vi "CH1_Comm.vi"() -> ()   [LabVIEW 2018]
uses:
  Stream/Stream.lvclass
  RxTx/RxTx.lvclass
  Stream/Stream.lvclass/Stream.ctl
panel:
  in  "IP: 2":string="200.131.64.49"
  in  "RxTx.lvclass":refnum<class "RxTx.lvclass">
  in  "Stream.lvclass":refnum<class "Stream.lvclass">
  in  "RxTx.lvclass 2":refnum<class "RxTx.lvclass">
  in  "Stream.lvclass 2":refnum<class "Stream.lvclass">
  in  "Channel:":u16=1
  in  "IP:":string="200.131.64.48"
  # "Channel 1 Stream Communication"
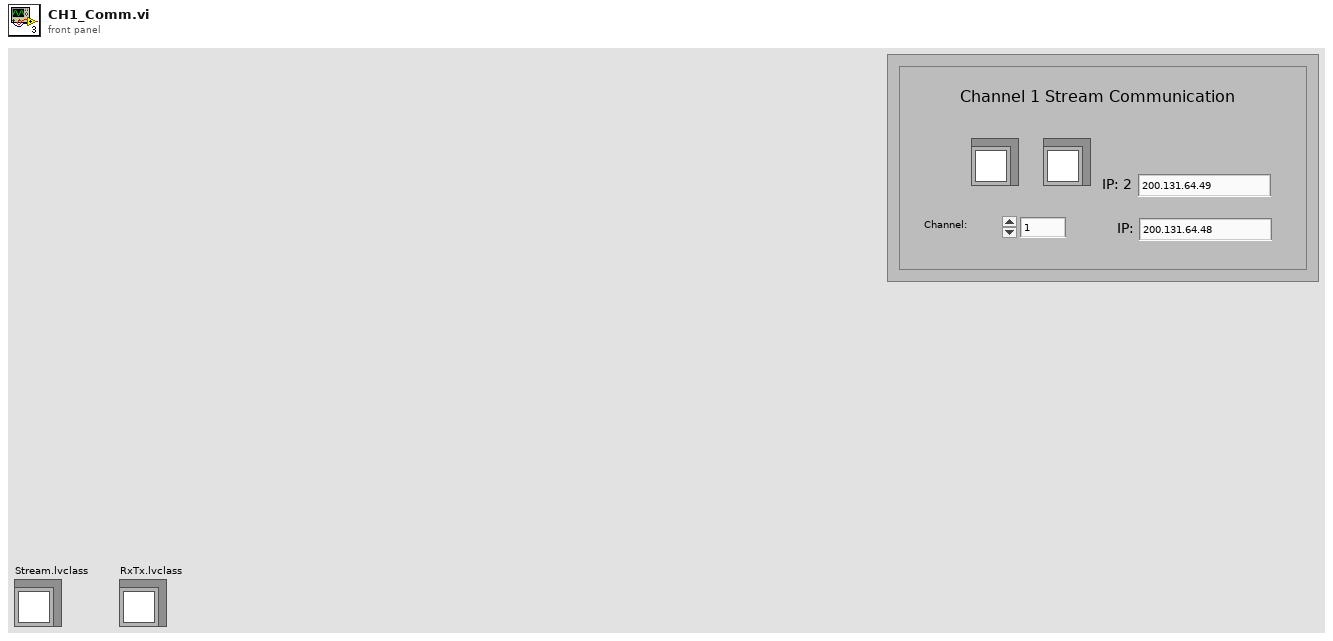
[diagram p1: front panel]
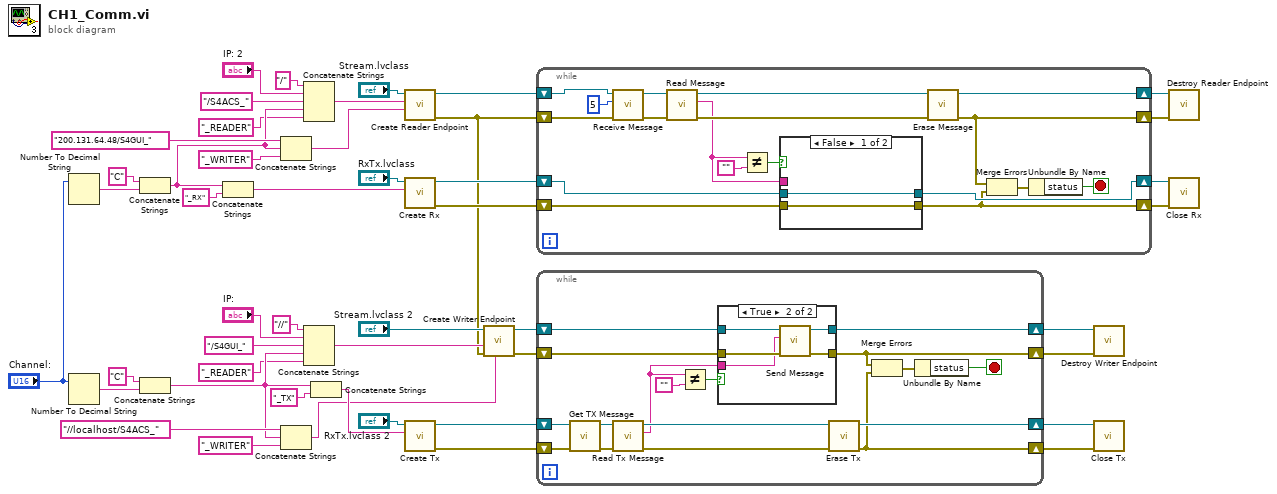
[diagram p0: block diagram]
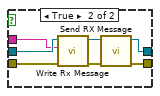
[diagram p2: hidden frame]
diagram:
  n1 = Number To Decimal String(number="Channel:") -> (decimal integer string=w15:string)  [unwired: 1 in]
  n2 = Number To Decimal String(number="Channel:") -> (decimal integer string=w34:string)  [unwired: 1 in]
  n3 = Concatenate Strings("C", w15) -> (w10:string)
  n4 = Concatenate Strings("C", w34) -> (w28:string)
  n5 = Concatenate Strings(w10, "_RX" ("Reader Name")) -> (w3:string)
  n6 = Concatenate Strings("200.131.64.48/S4GUI_" ("reader name"), w10, "_WRITER" ("reader name")) -> (w11:string)
  n7 = Concatenate Strings("//localhost/S4ACS_" ("reader name"), w28, "_WRITER" ("reader name")) -> (w29:string)
  n8 = Concatenate Strings("/" ("Reader Name"), "IP: 2", "/S4ACS_" ("Reader Name"), w10, "_READER" ("Reader Name")) -> (w8:string)
  n9 = Concatenate Strings("//" ("Reader Name"), "IP:", "/S4GUI_" ("Reader Name"), w28, "_READER" ("Reader Name")) -> (w26:string)
  n10 = Concatenate Strings(w28, "_TX" ("Reader Name")) -> (w32:string)
  n11 = call "Create Reader Endpoint.vi"("writer name"=w11, "reader name"=w8, "Stream in"="Stream.lvclass") -> ("error out"=w1:errorcluster, "Stream out"=w21:refnum<class "Stream.lvclass">)  [unwired: 7 in]
  n12 = call "Create Rx.vi"("Reader Name"=w3, "RxTx in"="RxTx.lvclass") -> ("error out"=w4:errorcluster, "RxTx out"=w5:refnum<class "RxTx.lvclass">)  [unwired: 8 in]
  n13 = call "Create Tx.vi"("Writer Name"=w32, "RxTx in"="RxTx.lvclass 2") -> ("error out"=w45:errorcluster, "RxTx out"=w46:refnum<class "RxTx.lvclass">)  [unwired: 8 in]
  n14 = call "Create Writer Endpoint.vi"("writer name"=w29, "error in (no error)"=w1, "reader name"=w26, "Stream in"="Stream.lvclass 2") -> ("error out"=w40:errorcluster, "Stream out"=w42:refnum<class "Stream.lvclass">)  [unwired: 6 in]
  n15 = while {
    shift-right: [w48] -> w19
    shift-left: w1 -> [w62]
    shift-right: [w51] -> w24
    shift-left: w21 -> [w63]
    shift-right: [w53] -> w22
    shift-left: w4 -> [w55]
    shift-right: [w54] -> w23
    shift-left: w5 -> [w56]
    stop <- w64 stop-if-true
    n16 = call "Receive Message.vi"("error in (no error)"=w62, "timeout ms"=5, "Stream in"=w63) -> ("error out"=w60:errorcluster, "Stream out"=w59:refnum<class "Stream.lvclass">)  [unwired: 7 in]
    n17 = call "Read Message.vi"("error in (no error)"=w60, "Stream in"=w59) -> ("error out"=w52:errorcluster, "Message"=w49:string, "Stream out"=w50:refnum<class "Stream.lvclass">)  [unwired: 7 in]
    n18 = Not Equal?(x=w49, y="") -> (x != y?=w58:bool)
    n19 = case shown="False" w58 {
      tunnel: w56 -> [w67 w74]
      tunnel: w55 -> [w66 w73]
      tunnel: [w67 w70] -> w54
      tunnel: [w66 w69] -> w53
      tunnel: w49 -> [_ w68]
      frame False {
      }
      frame True {
        n20 = call "Write Rx Message.vi"("error in (no error)"=w73, "Rx Message"=w68, "RxTx in"=w74) -> ("error out"=w72:errorcluster, "RxTx out"=w71:refnum<class "RxTx.lvclass">)  [unwired: 7 in]
        n21 = call "Send RX Message.vi"("error in (no error)"=w72, "RxTx in"=w71) -> ("error out"=w69:errorcluster, "RxTx out"=w70:refnum<class "RxTx.lvclass">)  [unwired: 8 in]
      }
    }
    n22 = call "Erase Message.vi"("error in (no error)"=w52, "Stream in"=w50) -> ("error out"=w48:errorcluster, "Stream out"=w51:refnum<class "Stream.lvclass">)  [unwired: 8 in]
    n23 = Merge Errors(w48, w53) -> (w65:errorcluster)
    n24 = Unbundle By Name(w65) -> ("status"=w64:bool)
  }
  n25 = while {
    shift-right: [w84] -> w39
    shift-left: w40 -> [w86]
    shift-right: [w85] -> w47
    shift-left: w42 -> [w87]
    shift-right: [w79] -> w43
    shift-left: w45 -> [w88]
    shift-right: [w81] -> w44
    shift-left: w46 -> [w89]
    stop <- w75 stop-if-true
    n26 = call "Get TX Message.vi"("error in (no error)"=w88, "RxTx in"=w89) -> ("error out"=w90:errorcluster, "RxTx out"=w77:refnum<class "RxTx.lvclass">)  [unwired: 8 in]
    n27 = call "Read Tx Message.vi"("error in (no error)"=w90, "RxTx in"=w77) -> ("error out"=w80:errorcluster, "Tx Message"=w76:string, "RxTx out"=w82:refnum<class "RxTx.lvclass">)  [unwired: 7 in]
    n28 = Not Equal?(x=w76, y="") -> (x != y?=w78:bool)
    n29 = case shown="True" w78 {
      tunnel: w87 -> [w93 w98]
      tunnel: w86 -> [w92 w97]
      tunnel: [w93 w96] -> w85
      tunnel: w76 -> [_ w95]
      tunnel: [w92 w94] -> w84
      frame False {
      }
      frame True {
        n30 = call "Send Message.vi"("error in (no error)"=w97, "Message"=w95, "Stream in"=w98) -> ("error out"=w94:errorcluster, "Stream out"=w96:refnum<class "Stream.lvclass">)  [unwired: 7 in]
      }
    }
    n31 = call "Erase Tx.vi"("error in (no error)"=w80, "RxTx in"=w82) -> ("error out"=w79:errorcluster, "RxTx out"=w81:refnum<class "RxTx.lvclass">)  [unwired: 8 in]
    n32 = Merge Errors(w84, w79) -> (w91:errorcluster)
    n33 = Unbundle By Name(w91) -> ("status"=w75:bool)
  }
  n34 = call "Destroy Writer Endpoint.vi"("error in (no error)"=w39, "Stream in"=w47) -> ()  [unwired: 8 in, 2 out]
  n35 = call "Close Tx.vi"("error in (no error)"=w43, "RxTx in"=w44) -> ()  [unwired: 8 in, 2 out]
  n36 = call "Destroy Reader Endpoint.vi"("error in (no error)"=w19, "Stream in"=w24) -> ()  [unwired: 8 in, 2 out]
  n37 = call "Close Rx.vi"("error in (no error)"=w22, "RxTx in"=w23) -> ()  [unwired: 8 in, 2 out]
